vi "WPI_MXP SPI Bus to first MXP Pin.vi"(7 "SPI Bus":T1) -> (8 "Shared MXP Pin":T2=enum."Invalid")   [LabVIEW 2017]
uses:
  <vilib>/Rock Robotics/WPI/MXP/WPI_MXP Shared MXP Pin.ctl
  <vilib>/Rock Robotics/SystemInterfaces/spilib/spi_bus.ctl
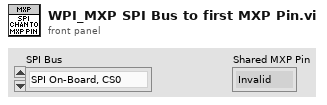
[diagram p1: front panel]
types:
  T1 = typedef "spi_bus.ctl" = enum16{"SPI On-Board, CS0", "SPI On-Board, CS1", "SPI On-Board, CS2", "SPI On-Board, CS3", "SPI MXP", "Invalid"}
  T2 = typedef "WPI_MXP Shared MXP Pin.ctl" = enum16{"11", "13", "15", "17", "19", "21", "23", "25", "27", "29", "31", "18", "22", "26", "32", "34", "Invalid"}
  T3 = enum16{"11", "13", "15", "17", "19", "21", "23", "25", "27", "29", "31", "18", "22", "26", "32", "34", "Invalid"}
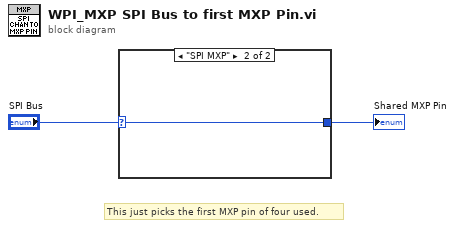
[diagram p0: block diagram]
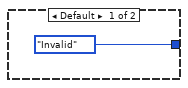
[diagram p2: hidden frame]
diagram:
  # "This just picks the first MXP pin of four used."
  n1 = case shown="\"SPI MXP\"" "SPI Bus" {
    selector: "SPI Bus" -> [_ w4]
    tunnel: [T3."Invalid" ("Shared MXP Pin") w4] -> w1
    frame Default {
    }
    frame "SPI MXP" {
    }
  }
  "Shared MXP Pin" <- w1
